vi "sensor_configurations.vi"() -> ()   [LabVIEW 2018]
uses:
  mono_config_camera.ctl
  mono_config_waypoint.ctl
  mono_config_sensor.ctl
  mono_config_radar.ctl
  mono_config_lidar.ctl
  mono_vehicle_config.ctl
panel:
  in  "vehicle":T1
  in  "lidar":T2
  in  "radar":T3
  in  "sensor":T4
  in  "waypoint":T5
  in  "camera":T6
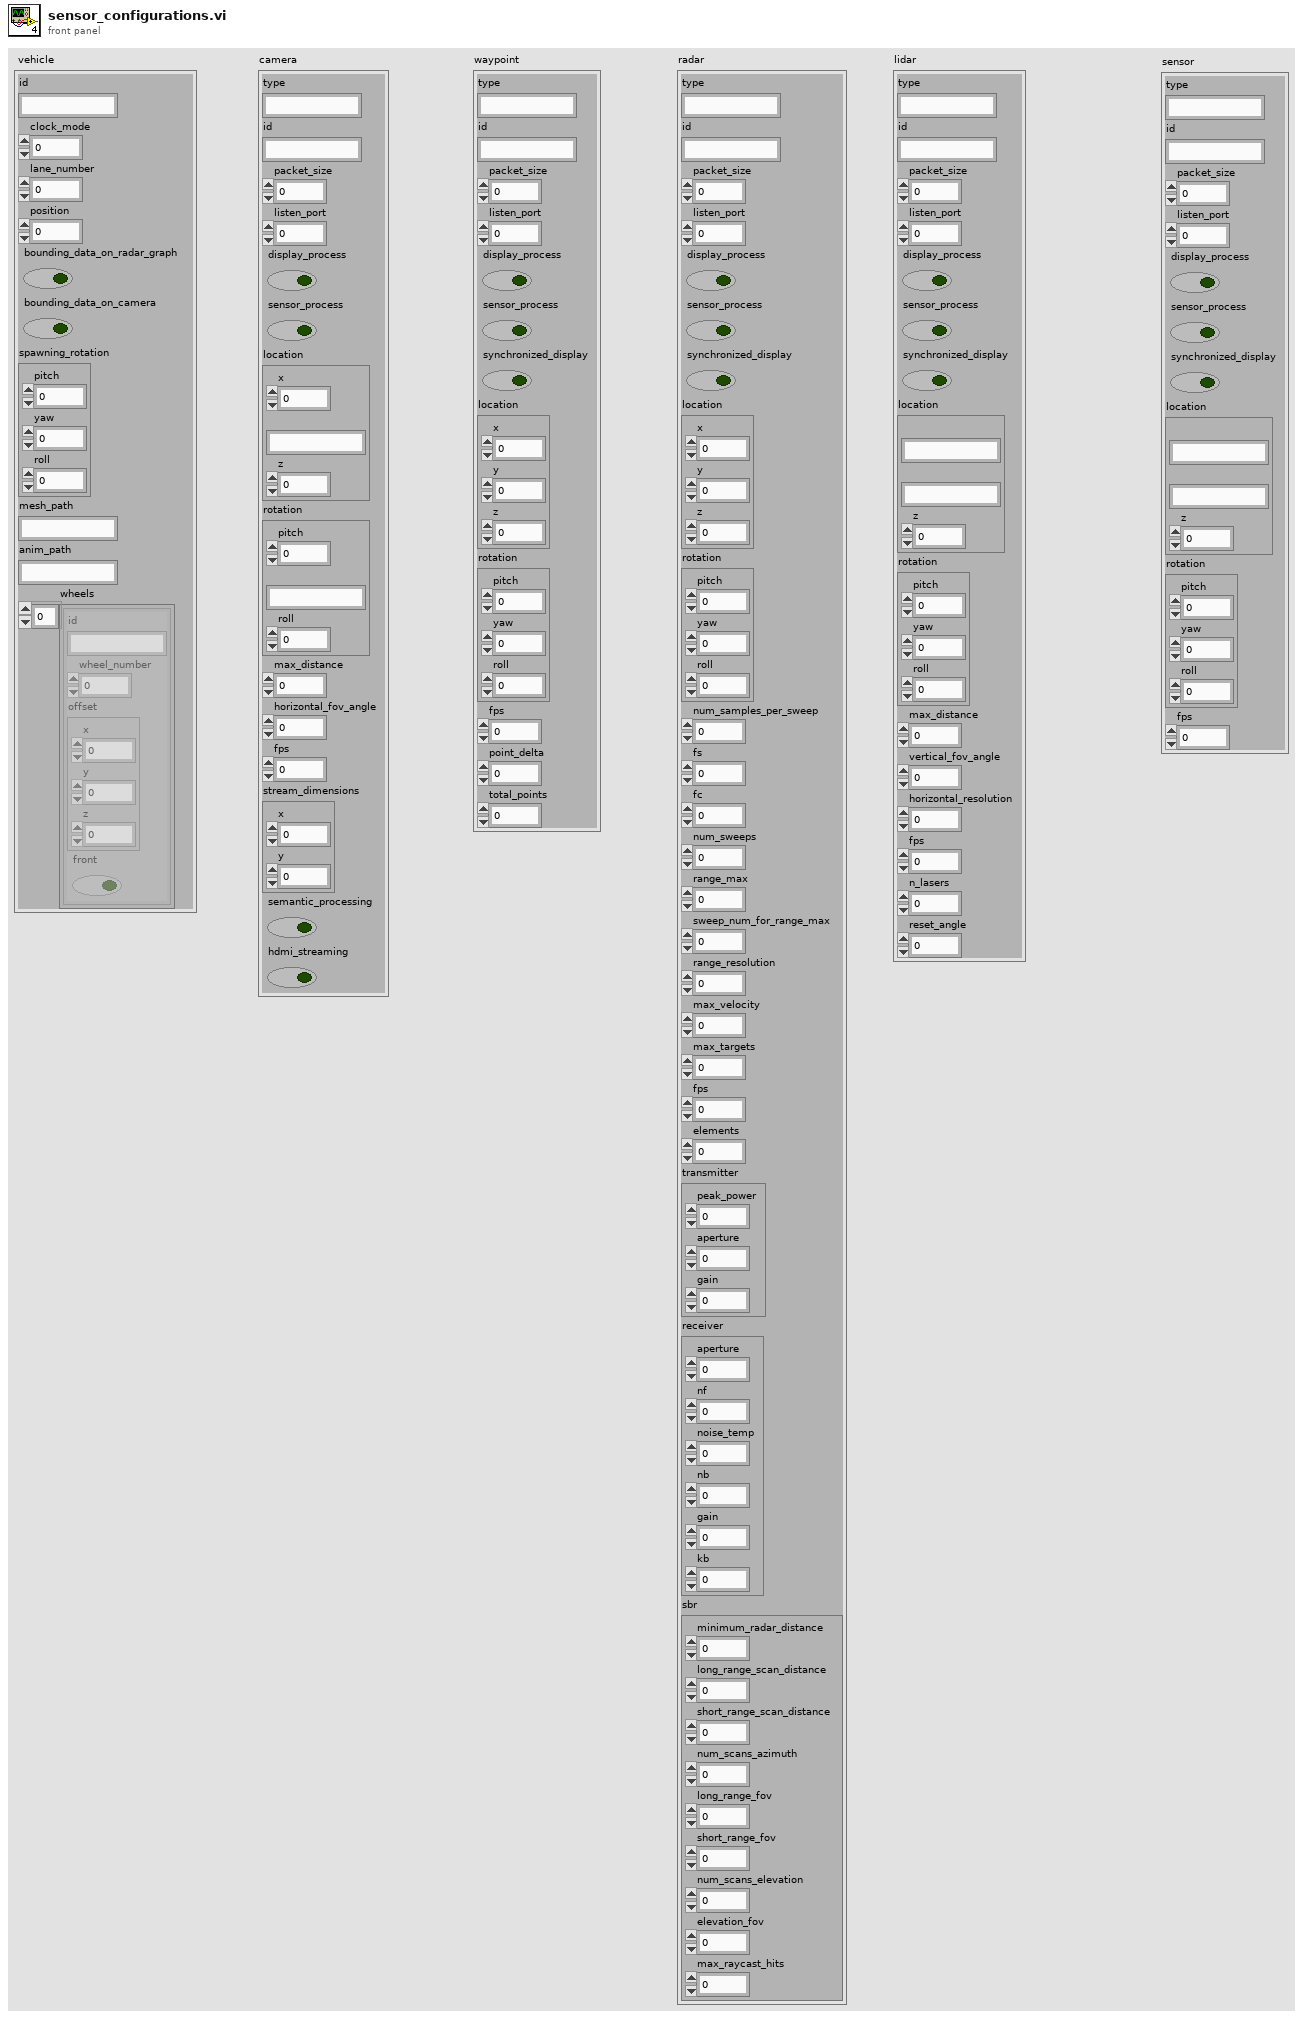
[diagram p1: front panel]
types:
  T1 = typedef "mono_vehicle_config.ctl" = cluster{"id":string, "clock_mode":i32, "lane_number":i32, "position":i32, "bounding_data_on_radar_graph":bool, "bounding_data_on_camera":bool, "spawning_rotation":cluster{"pitch":i32, "yaw":i32, "roll":i32}, "mesh_path":string, "anim_path":string, "wheels":cluster{"id":string, "wheel_number":i32, "offset":cluster{"x":i32, "y":i32, "z":i32}, "front":bool}[]}
  T2 = typedef "mono_config_lidar.ctl" = cluster{"type":string, "id":string, "packet_size":i32, "listen_port":i32, "display_process":bool, "sensor_process":bool, "synchronized_display":bool, "location":cluster{string, string, "z":i32}, "rotation":cluster{"pitch":i32, "yaw":i32, "roll":i32}, "max_distance":i32, "vertical_fov_angle":i32, "horizontal_resolution":i32, "fps":i32, "n_lasers":i32, "reset_angle":i32}
  T3 = typedef "mono_config_radar.ctl" = cluster{"type":string, "id":string, "packet_size":i32, "listen_port":i32, "display_process":bool, "sensor_process":bool, "synchronized_display":bool, "location":cluster{"x":i32, "y":i32, "z":i32}, "rotation":cluster{"pitch":i32, "yaw":i32, "roll":i32}, "num_samples_per_sweep":i32, "fs":i32, "fc":i32, "num_sweeps":i32, "range_max":i32, "sweep_num_for_range_max":i32, "range_resolution":i32, "max_velocity":i32, "max_targets":i32, "fps":i32, "elements":i32, "transmitter":cluster{"peak_power":i32, "aperture":i32, "gain":i32}, "receiver":cluster{"aperture":i32, "nf":i32, "noise_temp":i32, "nb":i32, "gain":i32, "kb":i32}, "sbr":cluster{"minimum_radar_distance":i32, "long_range_scan_distance":i32, "short_range_scan_distance":i32, "num_scans_azimuth":i32, "long_range_fov":i32, "short_range_fov":i32, "num_scans_elevation":i32, "elevation_fov":i32, "max_raycast_hits":i32}}
  T4 = typedef "mono_config_sensor.ctl" = cluster{"type":string, "id":string, "packet_size":i32, "listen_port":i32, "display_process":bool, "sensor_process":bool, "synchronized_display":bool, "location":cluster{string, string, "z":i32}, "rotation":cluster{"pitch":i32, "yaw":i32, "roll":i32}, "fps":i32}
  T5 = typedef "mono_config_waypoint.ctl" = cluster{"type":string, "id":string, "packet_size":i32, "listen_port":i32, "display_process":bool, "sensor_process":bool, "synchronized_display":bool, "location":cluster{"x":i32, "y":i32, "z":i32}, "rotation":cluster{"pitch":i32, "yaw":i32, "roll":i32}, "fps":i32, "point_delta":i32, "total_points":i32}
  T6 = typedef "mono_config_camera.ctl" = cluster{"type":string, "id":string, "packet_size":i32, "listen_port":i32, "display_process":bool, "sensor_process":bool, "location":cluster{"x":i32, string, "z":i32}, "rotation":cluster{"pitch":i32, string, "roll":i32}, "max_distance":i32, "horizontal_fov_angle":i32, "fps":i32, "stream_dimensions":cluster{"x":i32, "y":i32}, "semantic_processing":bool, "hdmi_streaming":bool}
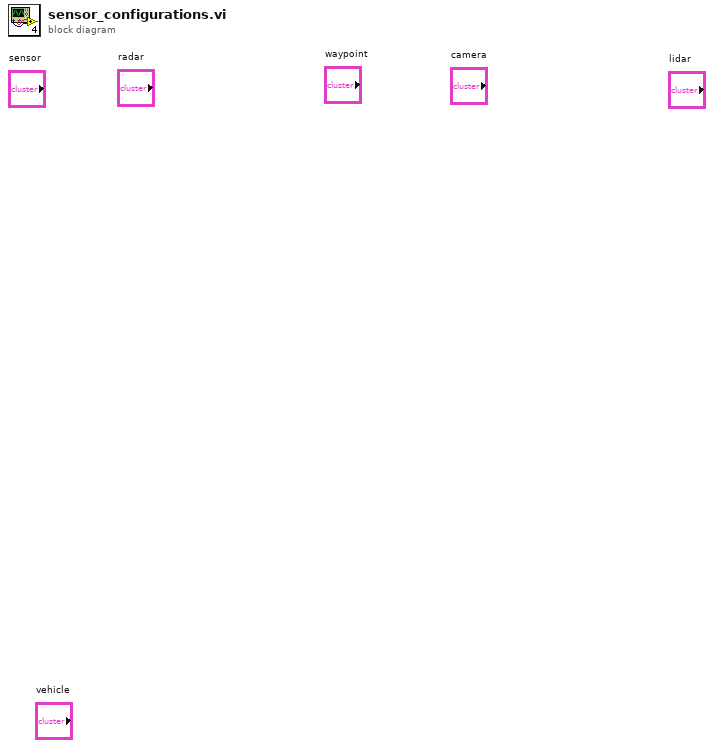
[diagram p0: block diagram]
diagram:
